vi "Invalid Lock.vi"(7 "source vi name":string, 8 "error in (no error)":errorcluster, 11 "Lockable Pointer in":refnum<class "Protected Pointer.lvclass">) -> (0 "error out":errorcluster, 3 "Lockable Pointer out":refnum<class "Protected Pointer.lvclass">)   [LabVIEW 2017, in "Memory Manager.lvlib" / "Protected Pointer.lvclass"]
uses:
  Protected Pointer.lvclass
  Errors.ctl
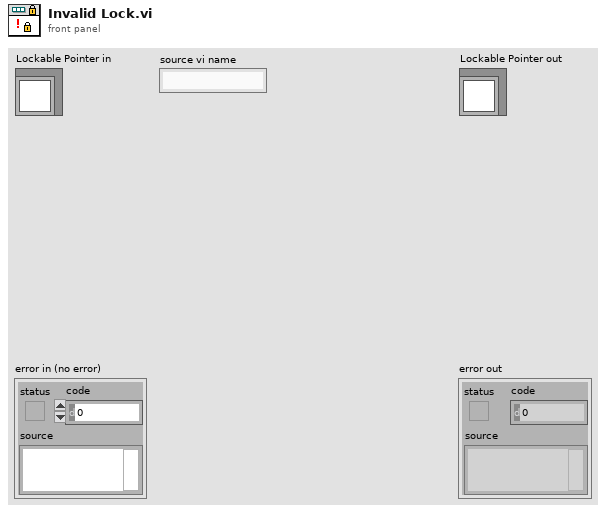
[diagram p1: front panel]
types:
  T1 = typedef "Memory Manager.lvlib/Protected Pointer.lvclass/Errors.ctl" = enum16{"Invalid Lock"}
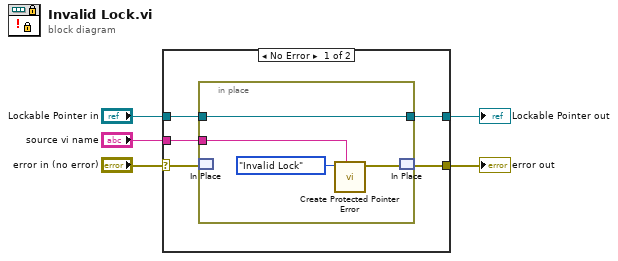
[diagram p0: block diagram]
diagram:
  n1 = case shown="No Error" "error in (no error)" {
    selector: "error in (no error)" -> [w10 w15]
    tunnel: [w9 w15] -> w4
    tunnel: "Lockable Pointer in" -> [w8 w16]
    tunnel: [w7 w16] -> w2
    tunnel: "source vi name" -> [w6 _]
    frame No Error {
      n2 = in-place {
        in-place-border: w8 -> [w13]
        in-place-border: [w13] -> w7
        in-place-border: w6 -> [w11]
        n3 = in-place-match #1(w10) -> ()  [unwired: 1 out]
        n4 = call "Create Protected Pointer Error.vi"("source vi name"=w11, "error"=Errors."Invalid Lock") -> ("error out"=w12:errorcluster)  [unwired: 8 in, 1 out]
        n5 = in-place-match #1(w12) -> (w9:errorcluster)
      }
    }
    frame Error {
    }
  }
  "error out" <- w4
  "Lockable Pointer out" <- w2
